vi "DAQNavi Read (Analog Wfm 1Chan 1Samp).vi"(8 "error in (no error)":errorcluster, 10 "timeout":dbl=10.0, 11 "task in":i32) -> (0 "error out":errorcluster, 2 "data":waveform(dbl), 3 "task out":i32)   [LabVIEW 2020]
uses:
  DAQNavi_LV.dll
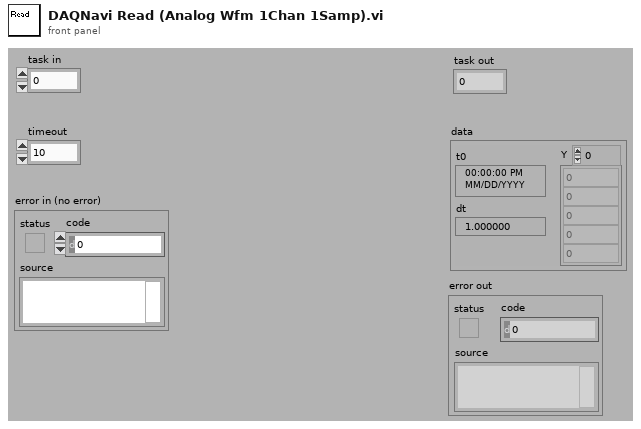
[diagram p1: front panel]
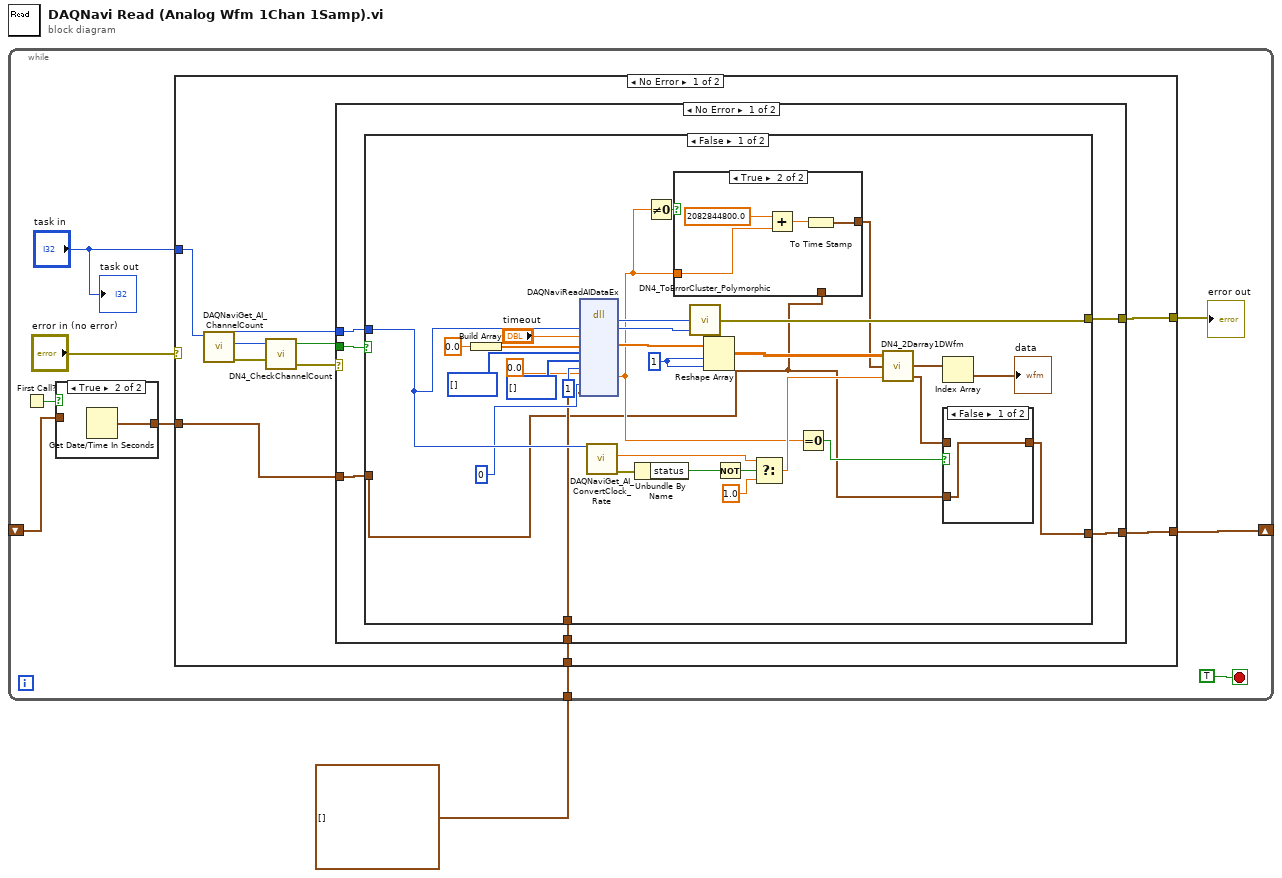
[diagram p0: block diagram]
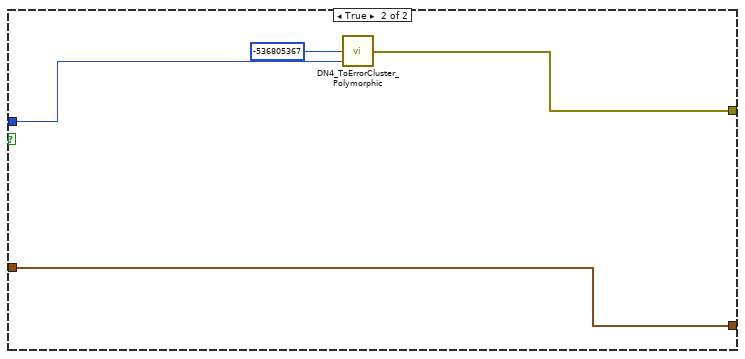
[diagram p5: hidden frame]
diagram:
  n1 = while {
    shift-right: [w3] -> _
    shift-left: _ -> [w5]
    tunnel: cluster{"Data Index":i64, "Src Id":i64}[] [] -> [w2]
    stop <- TRUE stop-if-true
    n2 = First Call?() -> (First Call?: T/F=w6:bool)
    n3 = case shown="True" w6 {
      tunnel: w5 -> [w11 _]
      tunnel: [w11 w12] -> w4
      frame False {
      }
      frame True {
        n4 = Get Date/Time In Seconds() -> (seconds since 1Jan1904=w12:timestamp)
      }
    }
    n5 = case shown="No Error" "error in (no error)" {
      selector: "error in (no error)" -> [_ w74]
      tunnel: "task in" -> [w22 _]
      tunnel: [w21 w74] -> w9
      tunnel: w4 -> [w15 w73]
      tunnel: [w14 w73] -> w3
      tunnel: w2 -> [w13 _]
      frame No Error {
        n6 = call "DAQNaviGet_AI_ChannelCount.vi"("task in"=w22) -> ("error out"=w19:errorcluster, "channel count"=w20:i32, "task out"=w16:i32)  [unwired: 1 in, 7 out]
        n7 = call "DN4_CheckChannelCount.vi"("error out"=w19, "channel count"=w20) -> ("error IO"=w17:errorcluster, "greater than 1?"=w18:bool)  [unwired: 2 out]
        n8 = case shown="No Error" w17 {
          selector: w17 -> [_ w72]
          tunnel: w18 -> [w28 _]
          tunnel: [w27 w72] -> w21
          tunnel: w16 -> [w26 _]
          tunnel: w15 -> [w25 w71]
          tunnel: [w24 w71] -> w14
          tunnel: w13 -> [w23 _]
          frame No Error {
            n9 = case shown="False" w28 {
              tunnel: [w52 w69] -> w27
              tunnel: w26 -> [w48 w68]
              tunnel: w25 -> [w30 w67]
              tunnel: [w35 w67] -> w24
              tunnel: w23 -> [w33 _]
              frame False {
                w50 = 1 ("dimension size")
                n10 = Build Array(0.0 ("element")) -> (w54:dbl[])
                n11 = dll-call lib="DAQNavi_LV.dll" fn="DAQNaviReadAIDataEx"("taskID"=w48, "timeout"="timeout", "scaledData"=w54, "rawData16"=u16[] [], "rawData32"=u32[] [], "samples"=u32 1, "startTime"=0.0, "markCount"=0, "markBuf"=w33) -> ("return type"=w53:i32, "taskID"=w39:i32, "scaledData"=w51:dbl[], "startTime"=w31:dbl)  [unwired: 4 in, 7 out]
                n12 = call "DAQNaviGet_AI_ConvertClock_Rate.vi"("task in"=w48) -> ("error out"=w47:errorcluster, "rate"=w44:dbl)  [unwired: 1 in, 8 out]
                n13 = Unbundle By Name(w47) -> ("status"=w45:bool)
                n14 = Not Equal To 0?(x=w31) -> (x != 0?=w32:bool)
                n15 = case shown="True" w32 {
                  tunnel: w31 -> [_ w66]
                  tunnel: [w62 w63] -> w29
                  tunnel: w30 -> [w62 _]
                  frame False {
                  }
                  frame True {
                    n16 = Add(x=2082844800.0, y=w66) -> (x+y=w64:dbl)
                    n17 = To Time Stamp(1:w64) -> (0:w63:timestamp)
                  }
                }
                n18 = call "DN4_ToErrorCluster_Polymorphic.vi"("task id"=w39, "error code"=w53) -> ("error out"=w52:errorcluster)  [unwired: 3 out]
                n19 = Reshape Array(w51, w50, w50) -> (w49:dbl[][])
                n20 = Not(x=w45) -> (.not. x?=w46:bool)
                n21 = Select(t=w44, s=w46, f=1.0) -> (s? t:f=w42:dbl)
                n22 = Equal To 0?(x=w31) -> (x = 0?=w37:bool)
                n23 = call "DN4_2Darray1DWfm.vi"("rate"=w42, "StartTime"=w29, "2D Array"=w49) -> ("EndTime"=w36:timestamp, "1D Wfm"=w41:waveform(dbl)[])  [unwired: 1 out]
                n24 = Index Array(array=w41) -> (element=→"data":waveform(dbl))  [unwired: 1 in]
                n25 = case shown="False" w37 {
                  tunnel: w30 -> [w60 _]
                  tunnel: w36 -> [_ w61]
                  tunnel: [w60 w61] -> w35
                  frame False {
                  }
                  frame True {
                  }
                }
              }
              frame True {
                n26 = call "DN4_ToErrorCluster_Polymorphic.vi"("task id"=w68, "error code"=-536805367 ("error code (0)")) -> ("error out"=w69:errorcluster)  [unwired: 3 out]
              }
            }
          }
          frame Error {
          }
        }
      }
      frame Error {
      }
    }
    "error out" <- w9
    "task out" <- "task in"
  }
